vi "Calculate Gas Water Heater Energy.vi"(6 "Total_1":dbl, 9 "HHV_1":dbl format="%#.4f", 10 "Gross Heating Value, Vol (Real, Dry) in":dbl=1000.0 min=900.0 max=2600.0 step=1.0 format="%#.4f", 11 "Totalizer":dbl) -> (0 "Q1":dbl format="%#.4f", 1 "Q2":dbl format="%#.4f", 2 "Qt":dbl format="%#.4f", 3 "Total Energy":string)   [LabVIEW 2019]
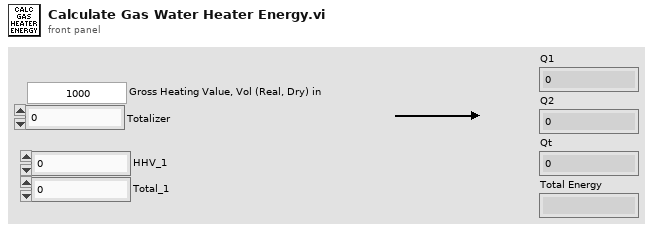
[diagram p1: front panel]
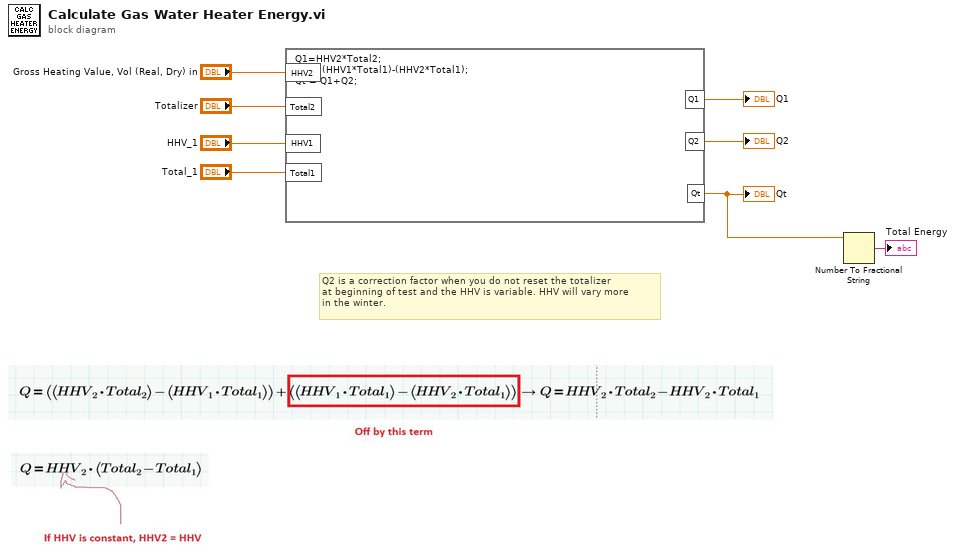
[diagram p0: block diagram]
diagram:
  # "Q2 is a correction factor when you do not reset the totalizer\nat beginning of test and the HHV is variable. HHV will vary more\nin the winter."
  n1 = formula code="Q1=HHV2*Total2;\nQ2 = (HHV1*Total1)-(HHV2*Total1);\nQt = Q1+Q2;"("Total2"="Totalizer", "HHV2"="Gross Heating Value, Vol (Real, Dry) in", "HHV1"="HHV_1", "Total1"="Total_1") -> ("Q1"=→"Q1":dbl, "Q2"=→"Q2":dbl, "Qt"=w1:dbl)
  "Qt" <- w1
  n2 = Number To Fractional String(number=w1) -> (F-format string=→"Total Energy":string)  [unwired: 3 in]
